vi "PMD Get Power.vi"(0 "VISA In":refnum<visa-resource-name>, 1 "Wavelength (nm)":dbl=100.0 min=0.0 max=2000.0 step=0.1 format="%.1f", 2 "Timeout (100 ms)":i32=100, 3 "error in":errorcluster) -> (4 "New":bool, 5 "PMD Error":string, 6 "VISA out":refnum<visa-resource-name>, 7 "Readout value":dbl format="%^#_9e", 8 "Readout string":string, 9 "error out":errorcluster)   [LabVIEW 2010]
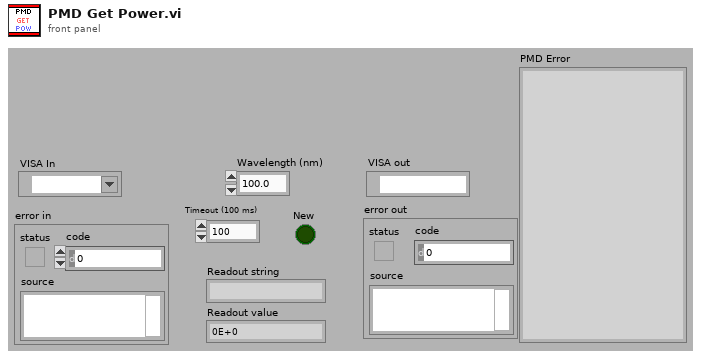
[diagram p1: front panel]
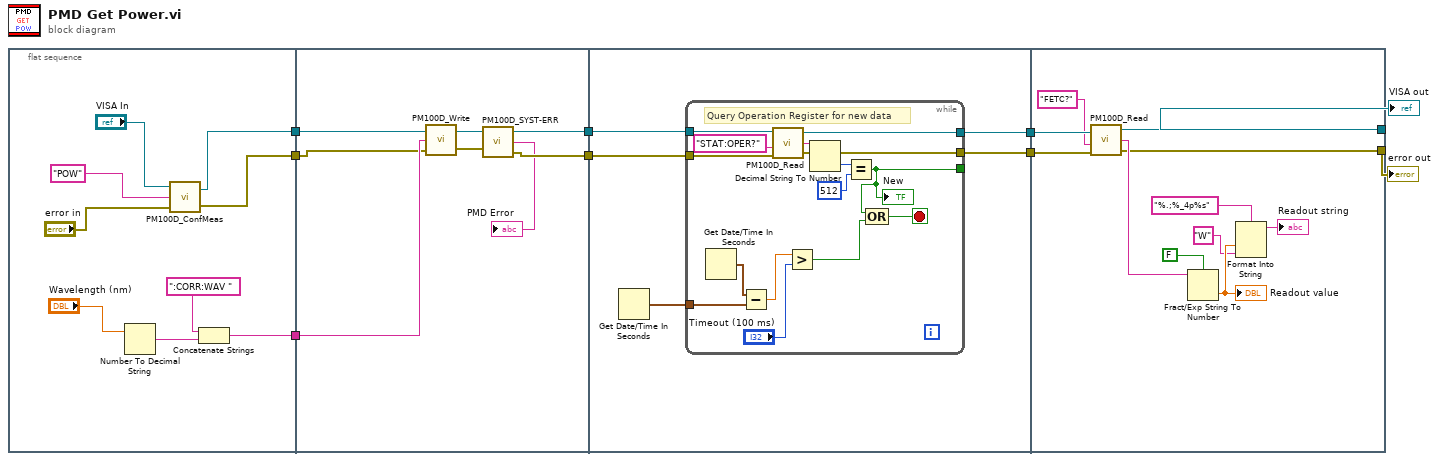
[diagram p0: block diagram]
diagram:
  n1 = flat-sequence {
    tunnel: [w17] -> w5
    tunnel: [w16] -> w3
    tunnel: [w10] -> w1
    tunnel: w5 -> [w25]
    tunnel: [w21] -> w4
    tunnel: w3 -> [w24]
    tunnel: [w20] -> w2
    tunnel: w1 -> [w26]
    tunnel: w4 -> [w31]
    tunnel: w2 -> [w30]
    tunnel: [w28] -> w9
    tunnel: [w27] -> w8
    tunnel: w9 -> [w57]
    tunnel: w8 -> [w56]
    tunnel: [w48] -> w6
    tunnel: [w47] -> w7
    frame #0 {
      n2 = Number To Decimal String(number="Wavelength (nm)") -> (decimal integer string=w12:string)  [unwired: 1 in]
      n3 = call "PM100D_ConfMeas.vi"("error in"="error in", "Conf:"="POW" ("Command"), "VISA In"="VISA In") -> ("error out"=w16:errorcluster, "dup VISA session"=w17:refnum<visa-resource-name>)
      n4 = Concatenate Strings(":CORR:WAV " ("string"), w12) -> (w10:string)
    }
    frame #1 {
      n5 = call "PM100D_Write.vi"("error in (no error)"=w24, "Command"=w26, "VISA in"=w25) -> ("error out"=w22:errorcluster, "VISA out"=w23:refnum<visa-resource-name>)
      n6 = call "PM100D_SYST-ERR.vi"("error out 2"=w22, "VISA In"=w23) -> ("error out"=w20:errorcluster, "Error"=→"PMD Error":string, "VISA Out"=w21:refnum<visa-resource-name>)  [unwired: 1 in]
    }
    frame #2 {
      n7 = Get Date/Time In Seconds() -> (seconds since 1Jan1904=w29:timestamp)
      n8 = while {
        tunnel: w31 -> [w42]
        tunnel: w30 -> [w41]
        tunnel: [w40] -> w28
        tunnel: [w39] -> w27
        tunnel: [w37] -> _
        tunnel: w29 -> [w35]
        stop <- w38 stop-if-true
        # "Query Operation Register for new data"
        n9 = Get Date/Time In Seconds() -> (seconds since 1Jan1904=w36:timestamp)
        n10 = Subtract(x=w36, y=w35) -> (x-y=w34:dbl)
        n11 = call "PM100D_Read.vi"("error in (no error)"=w41, "Command"="STAT:OPER?", "VISA in"=w42) -> ("error out"=w39:errorcluster, "ReadValue"=w45:string, "VISA out"=w40:refnum<visa-resource-name>)  [unwired: 1 in]
        n12 = Greater?(x=w34, y="Timeout (100 ms)") -> (0:w32:bool)
        n13 = Decimal String To Number(string=w45) -> (number=w44:i32)  [unwired: 2 in, 1 out]
        n14 = Equal?(x=w44, y=512) -> (x = y?=w37:bool)
        "New" <- w37
        n15 = Compound Arithmetic op=OR(w37, w32) -> (w38:bool)
      }
    }
    frame #3 {
      n16 = call "PM100D_Read.vi"("error in (no error)"=w56, "Command"="FETC?", "VISA in"=w57) -> ("error out"=w47:errorcluster, "ReadValue"=w49:string, "VISA out"=w48:refnum<visa-resource-name>)  [unwired: 1 in]
      n17 = Fract/Exp String To Number(use system decimal point (T)=FALSE, string=w49) -> (number=w52:dbl)  [unwired: 2 in, 1 out]
      "Readout value" <- w52
      n18 = Format Into String(format string="%.;%_4p%s", w52, "W") -> (resulting string=→"Readout string":string)  [unwired: 2 in, 1 out]
    }
  }
  "error out" <- w7
  "VISA out" <- w6
